vi "About Glimpse.vi"   [LabVIEW 2016]
uses:
  GLIMPSE Globals.vi
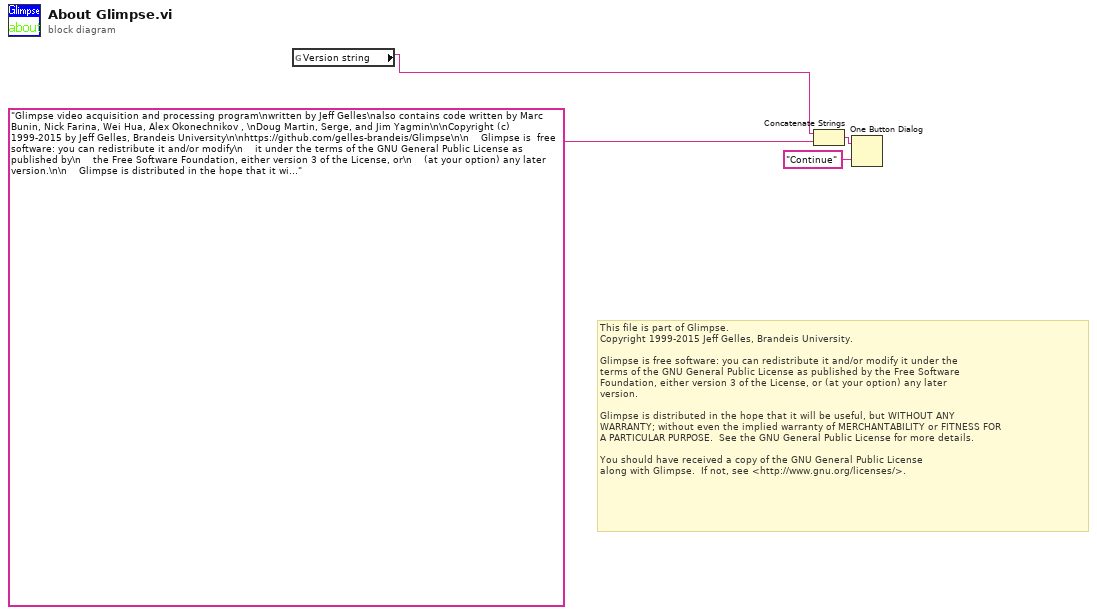
[diagram p0: block diagram]
diagram:
  # "This file is part of Glimpse. \nCopyright 1999-2015 Jeff Gelles, Brandeis University.    \n\nGlimpse is free software: you can redistribute it and/or modify it under the \nterms of the GNU General Public License as published by the Free Software \nFoundation, either version 3 of the License, or (at your option) any later \nversion.\n\nGlimpse is distributed in the hope that it will be useful, but WITHOUT ANY \nWARRANTY; without even the implied warranty of MERCHANTABILITY or FITNESS FOR \nA PARTICULAR PURPOSE.  See the GNU General Public License for more details.\n\nYou should have received a copy of the GNU General Public License\nalong with Glimpse.  If not, see <http://www.gnu.org/licenses/>."
  n1 = global read "GLIMPSE Globals.vi" "Version string"() -> (w1:string)
  n2 = Concatenate Strings(w1, "Glimpse video acquisition and processing program\nwritten by Jeff Gelles\nalso contains code written by Marc Bunin, Nick Farina, Wei Hua, Alex Okonechnikov , \nDoug Martin, Serge, and Jim Yagmin\n\nCopyright (c) 1999-2015 by Jeff Gelles, Brandeis University\n\nhttps://github.com/gelles-brandeis/Glimpse\n\n    Glimpse is  free software: you can redistribute it and/or modify\n    it under the terms of the GNU General Public License as published by\n    the Free Software Foundation, either version 3 of the License, or\n    (at your option) any later version.\n\n    Glimpse is distributed in the hope that it will be useful,\n    but WITHOUT ANY WARRANTY; without even the implied warranty of\n    MERCHANTABILITY or FITNESS FOR A PARTICULAR PURPOSE.  See the\n    GNU General Public License for more details.\n\n    You should have received a copy of the GNU General Public License\n    along with this program (see file gpl.txt).  If not, see <http://www.gnu.org/licenses/>.\n\n\nThe above license and copyright does not apply to the following subprograms:\n\nLev-Mar Fit to encoded 2D gaussian.vi\nGlimpse get new coefficients.vi\nLev-Mar abx with 2D encoded Gaussian.vi\nLev-Mar xx with 2D encoded Gaussian.vi\npartial derivative with 2D encoded guassian.vi\n\nThose subprograms are modifications of subprograms contained in the National Instruments \nLabView advanced analysis library.  The original subprograms are copyright National Instruments. " ("message")) -> (w3:string)
  n3 = One Button Dialog(message=w3, button name ("OK")="Continue") -> ()  [unwired: 1 out]
